vi "main.vi"() -> ()   [LabVIEW 2011, in "Run_protocols.lvclass"]
uses:
  Run_protocols.lvclass
  protocol_Logging/Protocol_Logging.lvclass
  protocol_Generic/Protocol_Generic.lvclass
  protocol_TwoCreep/Protocol_TwoCreep.lvclass
  protocol_MoveToSetpoint/Protocol_MoveToSetpoint.lvclass
panel:
  out "Protocol Names":string[](array[string])
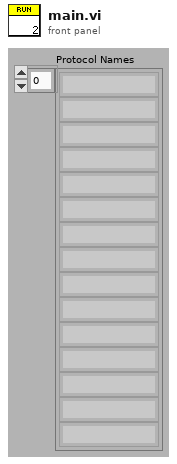
[diagram p1: front panel]
types:
  T1 = cluster{"Protocol_Logging.lvclass":refnum<class "Protocol_Logging.lvclass">, "Protocol_Generic.lvclass":refnum<class "Protocol_Generic.lvclass">, "Protocol_TwoCreep.lvclass":refnum<class "Protocol_TwoCreep.lvclass">, "Protocol_MoveToSetpoint.lvclass":refnum<class "Protocol_MoveToSetpoint.lvclass">}
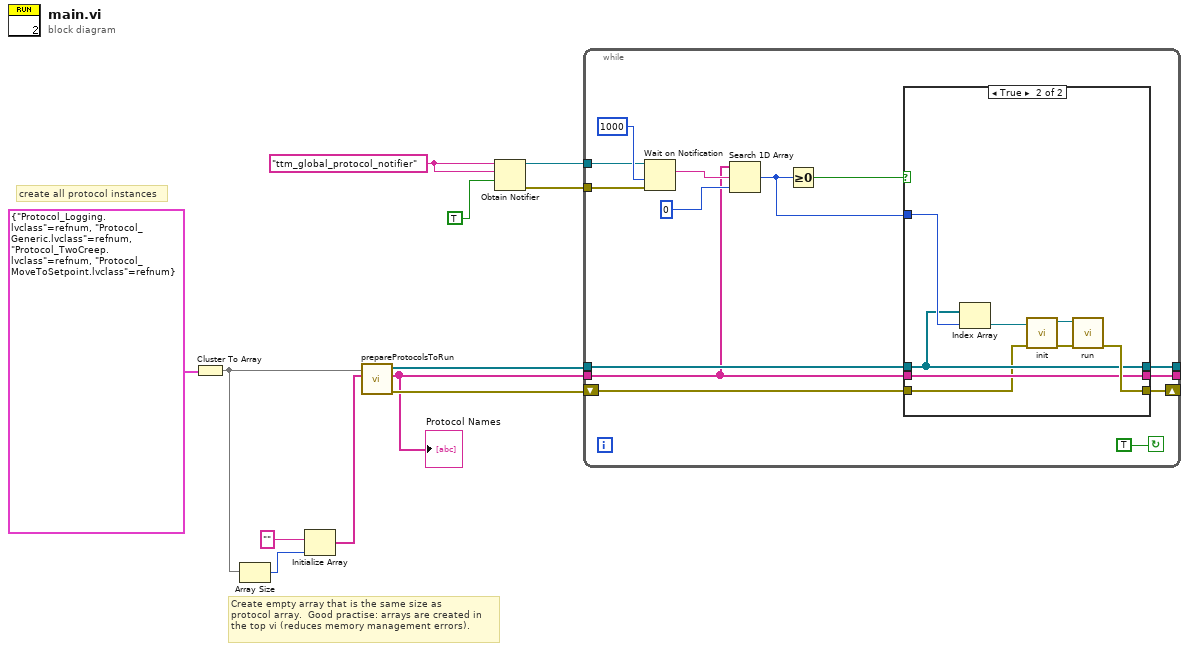
[diagram p0: block diagram]
diagram:
  w12 = "ttm_global_protocol_notifier" ("name (unnamed)")
  # "Create empty array that is the same size as \nprotocol array.  Good practise: arrays are created in\nthe top vi (reduces memory management errors)."
  # "create all protocol instances"
  n1 = Cluster To Array(cluster=T1 {"Protocol_Logging.lvclass"=refnum, "Protocol_Generic.lvclass"=refnum, "Protocol_TwoCreep.lvclass"=refnum, "Protocol_MoveToSetpoint.lvclass"=refnum}) -> (array=w2:refnum<class "Protocol_Generic.lvclass">[])
  n2 = Array Size(array=w2) -> (size(s)=w3:i32)
  n3 = Initialize Array("", w3) -> (w1:string[])
  n4 = call "prepareProtocolsToRun.vi"("protocolNameArrayIn"=w1, "protocolArray"=w2) -> ("errorOut"=w9:errorcluster, "protocolNameArrayOut"=w7:string[], "protocolArray"=w8:refnum<class "Protocol_Generic.lvclass">[])  [unwired: 7 in]
  "Protocol Names" <- w7
  n5 = Obtain Notifier(name (unnamed)=w12, notification data type=w12, create if not found? (T)=TRUE) -> (notifier out=w10:refnum<notifier>, error out=w6:errorcluster)  [unwired: 1 in, 1 out]
  n6 = while {
    tunnel: [w24] -> _
    tunnel: w10 -> [w23]
    tunnel: w8 -> [w20]
    tunnel: w7 -> [w14]
    shift-right: [w17] -> _
    shift-left: w9 -> [w16]
    tunnel: w6 -> [w15]
    tunnel: [w13] -> _
    stop <- TRUE continue-if-true
    n7 = Wait on Notification(notifier=w23, timeout in ms (-1)=1000, error in (no error)=w15) -> (notification=w22:string)  [unwired: 1 in, 3 out]
    n8 = Search 1D Array(1D array=w14, element=w22, start index (0)=0) -> (index of element=w18:i32)
    n9 = Greater Or Equal To 0?(x=w18) -> (x >= 0?=w19:bool)
    n10 = case shown="True" w19 {
      tunnel: w20 -> [w29 w35]
      tunnel: w16 -> [w28 w31]
      tunnel: [w28 w37] -> w17
      tunnel: [w29 w35] -> w24
      tunnel: w18 -> [_ w36]
      tunnel: w14 -> [w27 w34]
      tunnel: [w27 w34] -> w13
      frame False {
      }
      frame True {
        n11 = Index Array(array=w35, index=w36) -> (element=w33:refnum<class "Protocol_Generic.lvclass">)
        n12 = call-dynamic "init.vi"("error in (no error)"=w31, "Protocol_Generic in"=w33) -> ("error out"=w30:errorcluster, "Protocol_Generic out"=w32:refnum<class "Protocol_Generic.lvclass">)  [unwired: 8 in]
        n13 = call-dynamic "run.vi"("error in (no error)"=w30, "Protocol_Generic in"=w32) -> ("error out"=w37:errorcluster)  [unwired: 8 in, 1 out]
      }
    }
  }
